vi "Photobooth.vi"() -> ()   [LabVIEW 2012]
uses:
  <vilib>/userdefined/High Color/IMAQdx.ctl
  <vilib>/LVH/i3 Twitter/Controls/Twitter Handle.ctl
  <vilib>/LVH/i3 OAuth/Controls/OAuth Handle.ctl
  <vilib>/LVH/i3 OAuth/Controls/Signature Method.ctl
  <vilib>/LVH/i3 OAuth/Controls/Credentials.ctl
  Twitter/Twitter States.ctl
  Flickr API/Flickr States.ctl
  TypeDEF/Core Data.ctl
  <vilib>/vision/Image Controls.llb/IMAQ Image.ctl
  <vilib>/LVH/i3 Twitter/SubVIs/Twitter Open - Desktop.vi
  <vilib>/LVH/i3 Twitter/Tweets with Media/Post Media Tweet - From File.vi
  C:/Users/telsey/Desktop/Personal Projects/Photobooth/Flickr API/FlickrNet-3.5.0/FlickrNet.dll
  Flickr API/FlickrNet-3.5.0/FlickrNet.dll
  <vilib>/vision/driver/NI_Vision_Acquisition_Software.lvlib
  <vilib>/vision/NI_Vision_Development_Module.lvlib
  <vilib>/LVH/i3 Twitter/i3-twitter.lvlib
  <vilib>/LVH/i3 OAuth/i3-oauth.lvlib
panel:
  out "Snapshots":T1[](array[plugin-control])
  in  "Start Button":bool
  in  "Print":bool
  out "Timer":string
  out "Dial":u16(knob) max=100 scale=0.0..100.0
  out "Image":T1(plugin-control)
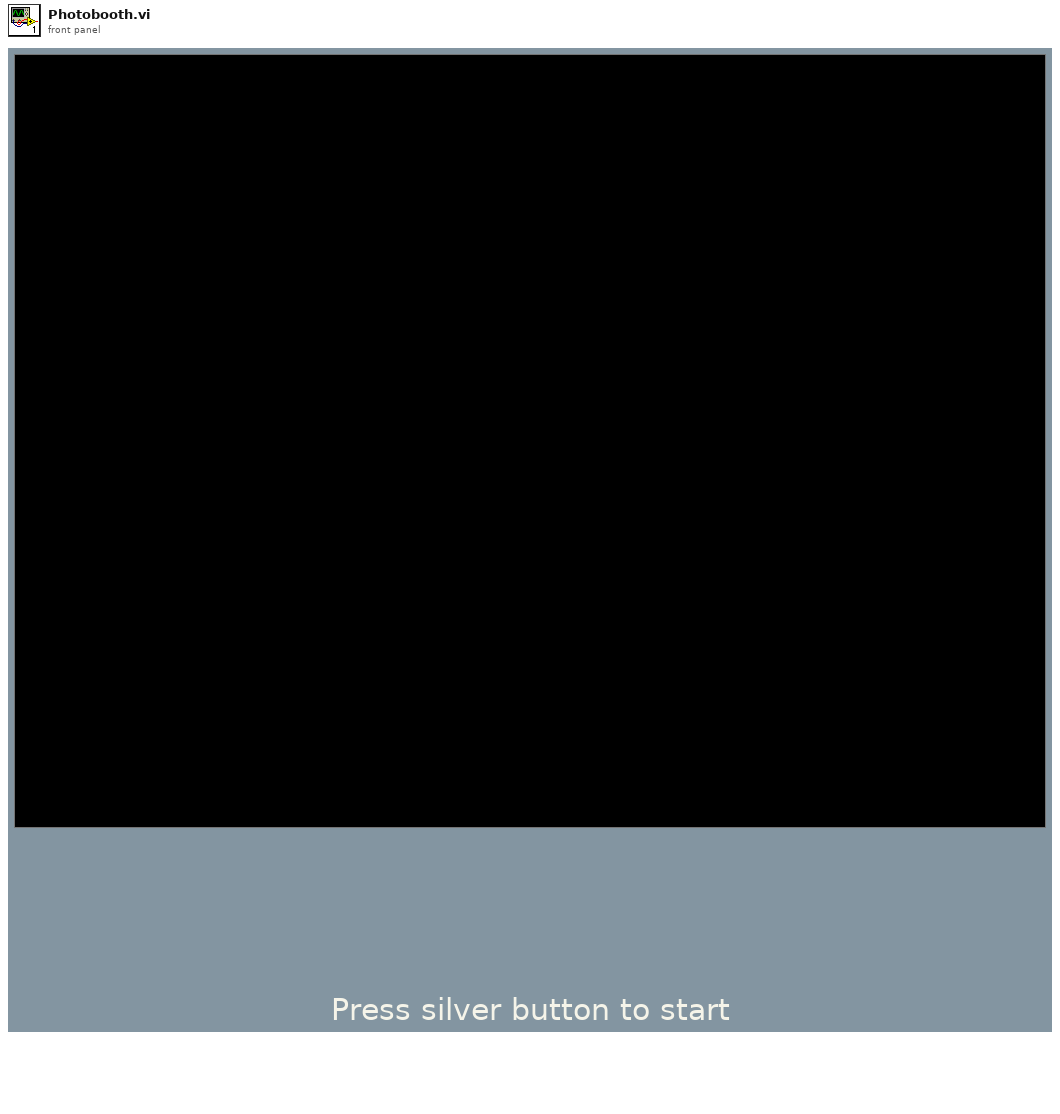
[diagram p1: front panel]
types:
  T1 = typedef "IMAQ Image.ctl" = refnum<image>
  T2 = typedef "Flickr States.ctl" = enum16{"Init", "Upload", "Close"}
  T3 = cluster{".Net Ref":refnum<k24>, "Init":cluster{"Enabled":bool, "Tag":string, "Photoset Name":string, "Photoset Description":string, "Album Cover":string}, "Path":path}
  T4 = typedef "Twitter States.ctl" = enum16{"Init", "Tweet", "Close"}
  T5 = typedef "i3-twitter.lvlib/Twitter Handle.ctl" = cluster{"OAuth Credentials":T6, "since ID":string, "max ID":string, "Screen Name":string}
  T6 = typedef "i3-oauth.lvlib/OAuth Handle.ctl" = cluster{"Signature Method":T7, "Version":string, "Client":T8, "Access":T8}
  T7 = typedef "i3-oauth.lvlib/Signature Method.ctl" = enum16{"HMAC-MD5", "HMAC-SHA1", "HMAC-SHA224", "HMAC-SHA256", "HMAC-SHA384", "HMAC-SHA512"}
  T8 = typedef "i3-oauth.lvlib/Credentials.ctl" = cluster{"Token":string, "Secret":string}
  T9 = cluster{"Handle":T5, "Access Credentials":T8, "Init":cluster{"Enabled":bool, "Tag":string}, "Image":path}
  T10 = typedef "IMAQdx.ctl" = refnum<k21>
  T11 = enum32{"invalid app kind", "Development System", "Run Time System", "Student Edition", "Embedded LabVIEW", "Evaluation", "Custom"}
  T12 = typedef "Core Data.ctl" = cluster{"Core":cluster{"Current VI Reference":refnum<vi>, "Close Panel on Exit?":bool}, "Camera":T10, "Images":T1[], "Current Image":u8, "Video Queue":refnum<queue>, "Wait":u8[], "Images Folder":path, "Photoset done":bool, "Flickr Q":refnum<queue>, "Twitter Q":refnum<queue>}
  T13 = enum32{"Invalid", "Standard", "Closed", "Hidden", "Minimized", "Maximized"}
  T14 = cluster{"Current VI Reference":refnum<vi>, "Close Panel on Exit?":bool}
  T15 = cluster{"Enabled":bool, "Tag":string, "Photoset Name":string, "Photoset Description":string, "Album Cover":string}
  T16 = cluster{"Header":path, "Image Folder":path, "Background":u32}
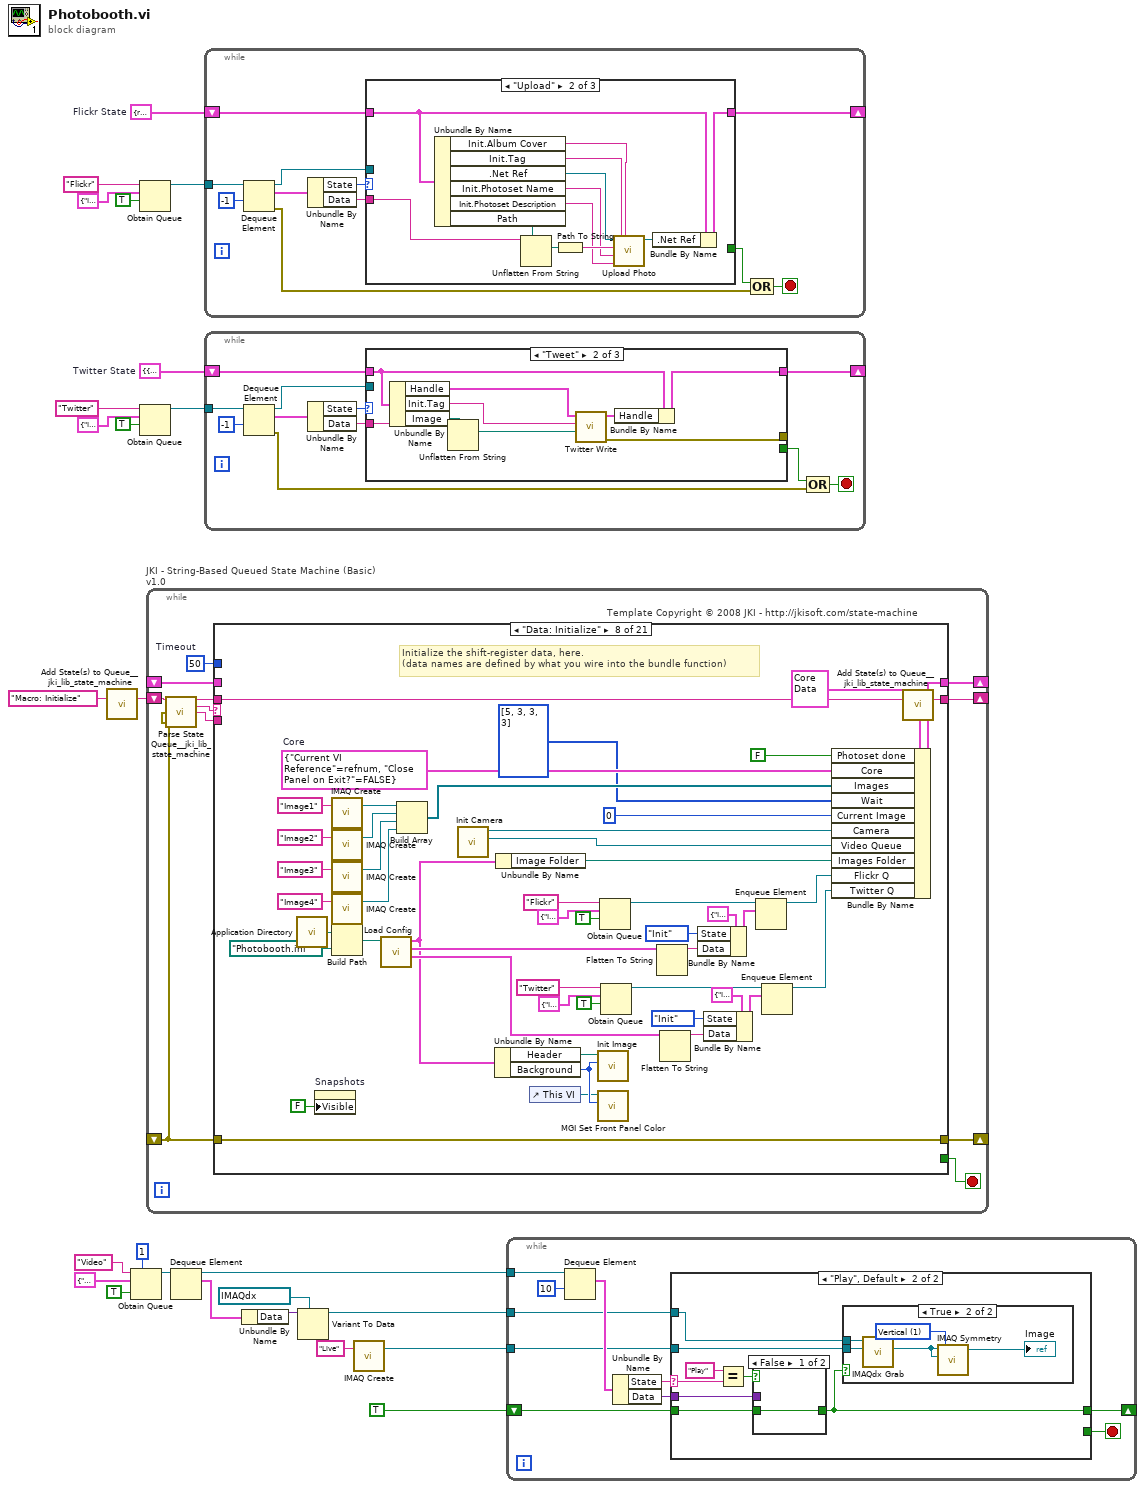
[diagram p0: block diagram]
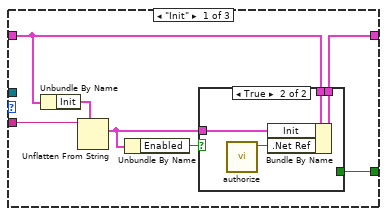
[diagram p2: hidden frame]
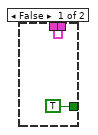
[diagram p3: hidden frame]
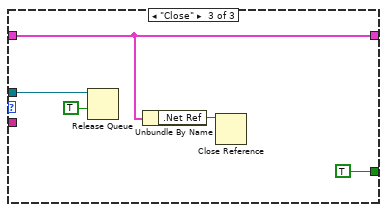
[diagram p4: hidden frame]
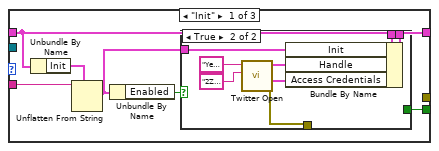
[diagram p5: hidden frame]
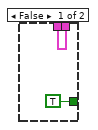
[diagram p6: hidden frame]
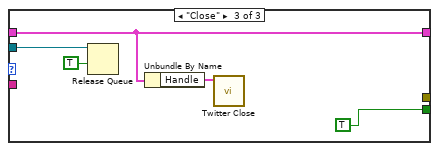
[diagram p7: hidden frame]
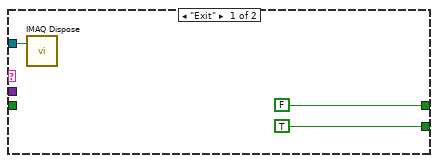
[diagram p8: hidden frame]
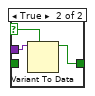
[diagram p9: hidden frame]
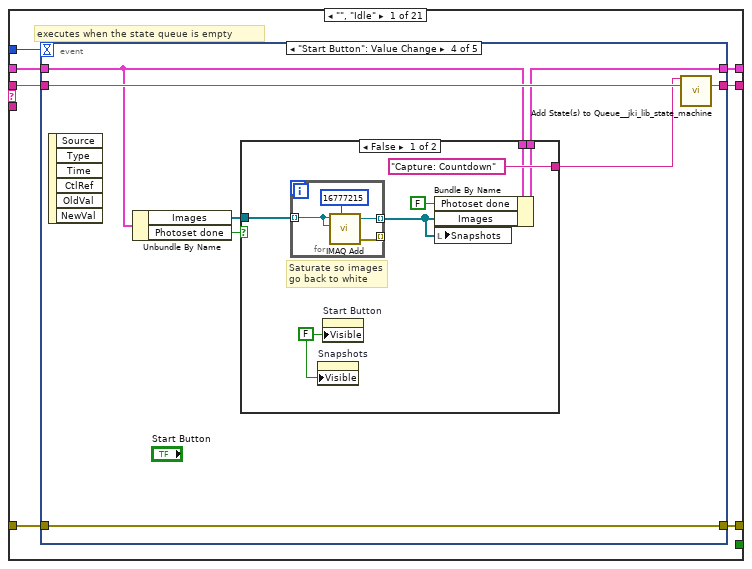
[diagram p11: hidden frame]
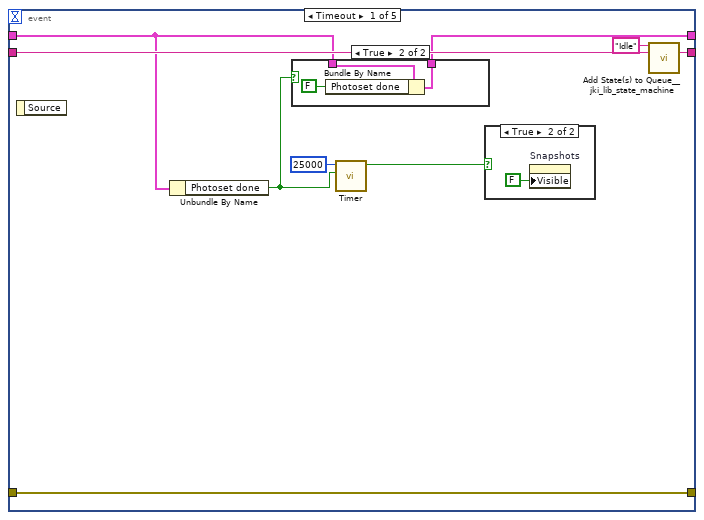
[diagram p12: hidden frame]
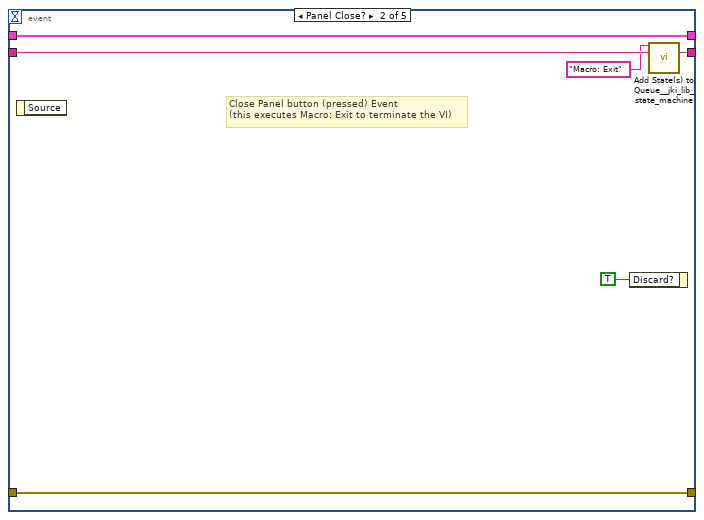
[diagram p15: hidden frame]
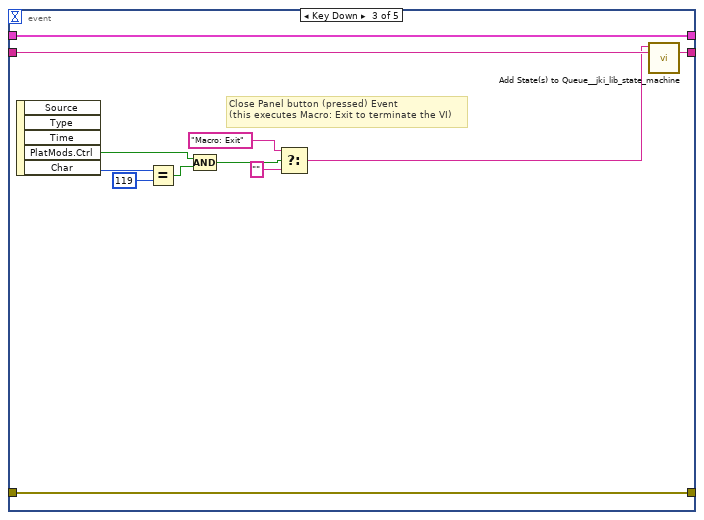
[diagram p16: hidden frame]
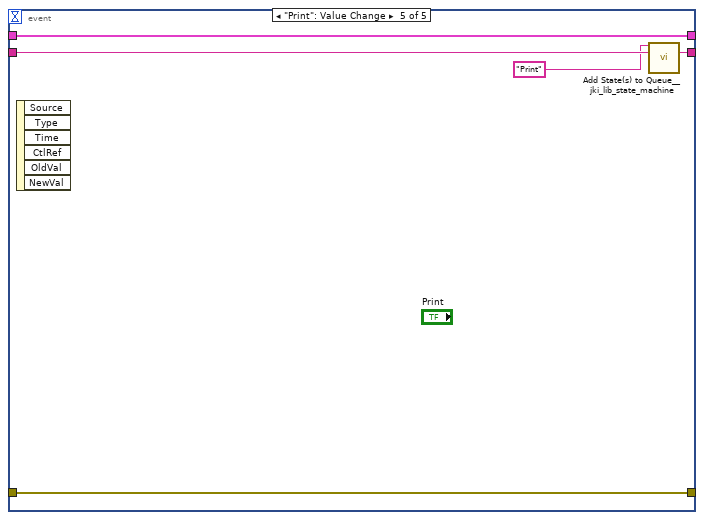
[diagram p18: hidden frame]
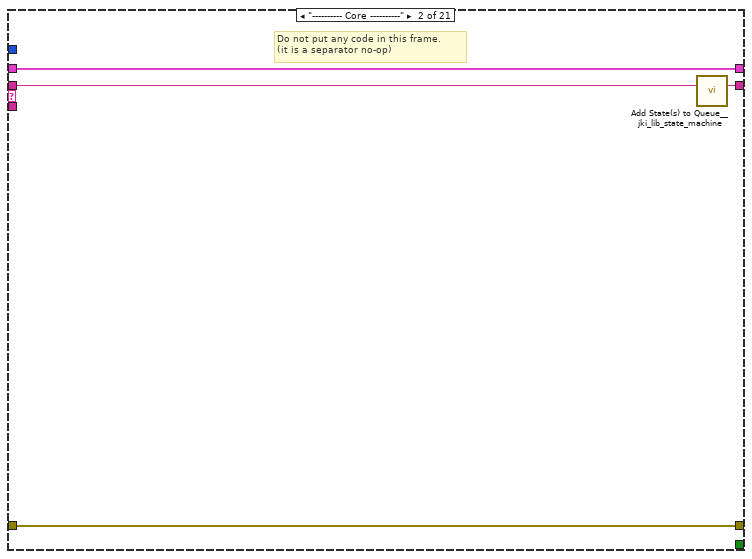
[diagram p19: hidden frame]
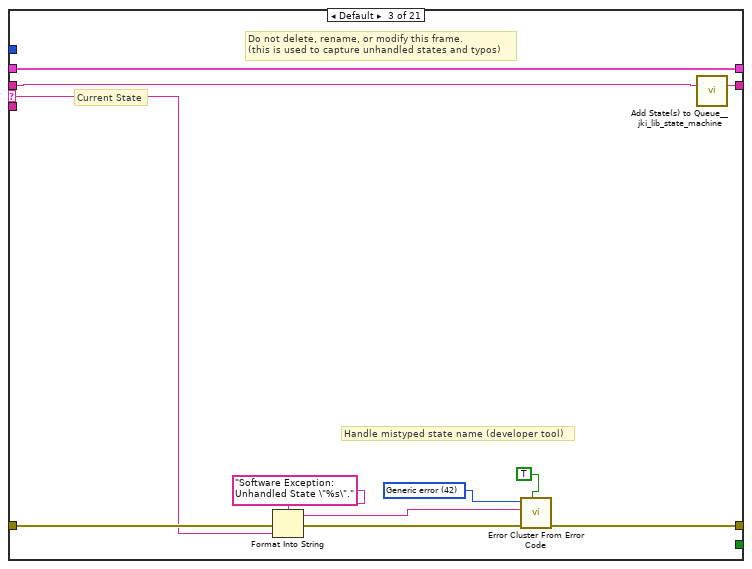
[diagram p20: hidden frame]
diagram:
  w5 = T3 {".Net Ref"=refnum, "Init"={"Enabled"=FALSE, "Tag"="", "Photoset Name"="", "Photoset Description"="", "Album Cover"=""}, "Path"=path ""}  # Flickr State
  w6 = T9 {"Handle"={"OAuth Credentials"={"Signature Method"=enum."HMAC-SHA1", "Version"="1.0", "Client"={"Token"="", "Secret"=""}, "Access"={"Token"="", "Secret"=""}}, "since ID"="", "max ID"="", "Screen Name"=""}, "Access Credentials"={"Token"="", "Secret"=""}, "Init"={"Enabled"=FALSE, "Tag"=""}, "Image"=path ""}  # Twitter State
  n1 = call <vilib>:"Add State(s) to Queue__jki_lib_state_machine.vi"("State(s) in (\"\")"="Macro: Initialize") -> ("States Out"=w25:string)  [unwired: 14 in]
  n2 = Obtain Queue(max queue size (-1, unlimited)=1, name (unnamed)="Video", element data type=cluster{"State":string, "Data":variant} {"State"="", "Data"=variant} ("State Cluster"), create if not found? (T)=TRUE) -> (queue out=w22:refnum<queue>)  [unwired: 1 in, 2 out]
  n3 = Obtain Queue(name (unnamed)="Flickr", element data type=cluster{"State":T2, "Data":string} {"State"=enum."Init", "Data"=""} ("name (unnamed)"), create if not found? (T)=TRUE) -> (queue out=w1:refnum<queue>)  [unwired: 2 in, 2 out]
  n4 = Obtain Queue(name (unnamed)="Twitter", element data type=cluster{"State":T4, "Data":string} {"State"=enum."Init", "Data"=""} ("name (unnamed)"), create if not found? (T)=TRUE) -> (queue out=w10:refnum<queue>)  [unwired: 2 in, 2 out]
  n5 = while "JKI - String-Based Queued State Machine (Basic) v1.0" {
    shift-right: [w29] -> _
    shift-left: _ -> [w28]
    shift-right: [w32] -> _
    shift-left: _ -> [w26]
    shift-right: [w31] -> _
    shift-left: w25 -> [w33]
    stop <- w30 stop-if-true
    w27 = 50  # Timeout
    # "Template Copyright © 2008 JKI - http://jkisoft.com/state-machine"
    n6 = call <vilib>:"Parse State Queue__jki_lib_state_machine.vi"("State Queue"=w33, "Error In (no error)"=w26) -> ("Remaining States"=w35:string, "Current State"=w36:string, "Arguments"=w34:string)  [unwired: 11 in]
    n7 = case shown="\"Data: Initialize\"" w36 {
      selector: w36 -> [_ _ w105 _ _ _ _ _ _ _ _ _ _ _ _ _ _ _ _ _ _]
      tunnel: w35 -> [w43 w104 w109 w127 w133 w138 w142 w191 w215 w224 w235 w241 w252 w278 w283 w293 w297 w315 w326 w350 w382]
      tunnel: w34 -> [_ _ _ _ _ _ _ _ _ _ _ w236 w246 _ _ _ _ _ _ _ _]
      tunnel: w28 -> [w41 w101 w107 w118 w130 w136 w139 _ w211 w221 w226 w239 w248 w275 w280 w290 w294 w310 w323 w343 w378]
      tunnel: [w40 w102 w111 w124 errorcluster {"status"=FALSE, "code"=0, "source"=""} ("error out") w135 w140 w188 w212 w222 w233 w237 w249 w276 w281 w291 w295 w313 w324 w348 w380] -> w32
      tunnel: w26 -> [w39 w102 w110 w124 w129 w135 w140 w188 _ w222 w233 w238 w250 w276 w281 w291 w295 w313 w324 w348 w380]
      tunnel: [w42 w103 w108 w126 w132 w137 w141 w190 w214 w223 w234 w240 w251 w277 w282 w292 w296 w314 w325 w349 w381] -> w31
      tunnel: [_ _ _ _ _ TRUE _ _ _ _ _ _ _ _ _ _ _ _ _ _ _] -> w30
      tunnel: [w38 w101 w107 w125 w130 w136 w139 w189 w211 w221 w226 w239 w248 w275 w280 w290 w294 w310 w323 w343 w377] -> w29
      tunnel: w27 -> [w37 _ _ _ _ _ _ _ _ _ _ _ _ _ _ _ _ _ _ _ _]
      frame "", "Idle" {
        # "executes when the state queue is empty"
        n8 = event shown="[3] \"Start Button\": Value Change" {
          selector: _ -> [_ _ _ _ _]
          dyn-events: _ -> [_ _ _ _ _]
          timeout: w37 -> [_ _ _ _ _]
          tunnel: w43 -> [w52 w63 w75 w83 w100]
          tunnel: [w51 w62 w74 w82 w99] -> w42
          tunnel: w41 -> [w45 w60 w72 w78 w96]
          tunnel: [w50 w61 w73 w81 w98] -> w40
          tunnel: w39 -> [w50 w61 w73 w81 w98]
          tunnel: [w44 w60 w72 w77 w96] -> w38
          event Timeout {
            n9 = event-data() -> ()  [unwired: 1 in, 1 out]
            n10 = Unbundle By Name(w45) -> ("Photoset done"=w46:bool)
            n11 = case shown="True" w46 {
              tunnel: w45 -> [w53 w56]
              tunnel: [w53 w55] -> w44
              frame False {
              }
              frame True {
                n12 = Bundle By Name(cluster=w56, "Photoset done"=FALSE) -> (w55:T12)
              }
            }
            n13 = call "Timer.vi"("Reset?"=w46, "Time Limit (ms)"=u32 25000 ("Time Limit")) -> ("Elapsed?"=w47:bool)  [unwired: 8 in, 1 out]
            n14 = case shown="True" w47 {
              frame False {
              }
              frame True {
                n15 = property on="Snapshots" class="Arr (strict)"("Visible"=FALSE) -> ()  [unwired: 2 in, 2 out]
              }
            }
            n16 = call <vilib>:"Add State(s) to Queue__jki_lib_state_machine.vi"("State(s) in Front (\"\")"="Idle" ("State(s) in Front (\"\")"), "State(s) in (\"\")"=w52) -> ("States Out"=w51:string)  [unwired: 13 in]
          }
          event Panel Close? {
            # "Close Panel button (pressed) Event\n(this executes Macro: Exit to terminate the VI)"
            n17 = event-data() -> ()  [unwired: 1 in, 1 out]
            n18 = event-data("Discard?"=TRUE) -> ()  [unwired: 1 in, 1 out]
            n19 = call <vilib>:"Add State(s) to Queue__jki_lib_state_machine.vi"("State(s) in Front (\"\")"="Macro: Exit", "State(s) in (\"\")"=w63) -> ("States Out"=w62:string)  [unwired: 13 in]
          }
          event Key Down {
            # "Close Panel button (pressed) Event\n(this executes Macro: Exit to terminate the VI)"
            n20 = event-data() -> ("PlatMods.Ctrl"=w68:bool, "Char"=w71:i16)  [unwired: 1 in, 3 out]
            n21 = Equal?(x=w71, y=i16 119) -> (x = y?=w69:bool)
            n22 = Compound Arithmetic op=AND(w68, w69) -> (w67:bool)
            n23 = Select(t="Macro: Exit", s=w67, f="") -> (s? t:f=w65:string)
            n24 = call <vilib>:"Add State(s) to Queue__jki_lib_state_machine.vi"("State(s) in Front (\"\")"=w65, "State(s) in (\"\")"=w75) -> ("States Out"=w74:string)  [unwired: 13 in]
          }
          event "Start Button": Value Change {
            n25 = event-data() -> ()  [unwired: 1 in, 6 out]
            n26 = Unbundle By Name(w78) -> ("Images"=w79:T1[], "Photoset done"=w76:bool)
            n27 = case shown="False" w76 {
              tunnel: ["Capture: Countdown" _] -> w80
              tunnel: w79 -> [w89 _]
              tunnel: w78 -> [w88 w95]
              tunnel: [w87 w95] -> w77
              frame False {
                w85 = FALSE ("Visible")
                # "Saturate so images\ngo back to white"
                n28 = for {
                  tunnel: w89 -> [w94] mode=indexing
                  tunnel: [w92] -> w86 mode=indexing
                  tunnel: [w91] -> _ mode=indexing
                  n29 = call "IMAQ Add"("Image Src A"=w94, "Constant"=16777215, "Image Dst"=w94) -> ("Image Dst Out"=w92:T1, "error out"=w91:errorcluster)  [unwired: 4 in]
                }
                n30 = property on="Snapshots" class="Arr (strict)"("Visible"=w85) -> ()  [unwired: 2 in, 2 out]
                n31 = property on="Start Button" class="Bool"("Visible"=w85) -> ()  [unwired: 2 in, 2 out]
                n32 = Bundle By Name(cluster=w88, "Photoset done"=FALSE, "Images"=w86) -> (w87:T12)
                n33 = local write "Snapshots"(w86) -> ()
              }
              frame True {
              }
            }
            n34 = call <vilib>:"Add State(s) to Queue__jki_lib_state_machine.vi"("State(s) in Front (\"\")"=w80, "State(s) in (\"\")"=w83) -> ("States Out"=w82:string)  [unwired: 13 in]
          }
          event "Print": Value Change {
            n35 = event-data() -> ()  [unwired: 1 in, 6 out]
            n36 = call <vilib>:"Add State(s) to Queue__jki_lib_state_machine.vi"("State(s) in Front (\"\")"="Print", "State(s) in (\"\")"=w100) -> ("States Out"=w99:string)  [unwired: 13 in]
          }
        }
      }
      frame "---------- Core ----------" {
        # "Do not put any code in this frame.\n(it is a separator no-op)"
        n37 = call <vilib>:"Add State(s) to Queue__jki_lib_state_machine.vi"("State(s) in (\"\")"=w104) -> ("States Out"=w103:string)  [unwired: 14 in]
      }
      frame Default {
        w114 = 42 items=["No error", "Argument error", "Memory is full", "Out of zone", "End of file", "File already open", "Generic file I/O error", "File not found", "File permission error", "Disk is full", "Duplicate path", "Too many files open", "System feature not enabled", "Resource file not found", "Cannot add resource", "Resource not found", "Image not found", "Image memory error", "Pen does not exist", "Config type invalid", "Config token not found", "Config parse error", "Config memory error", "Bad external code format", "Bad external code offset", "External code not present", "Null window", "Destroy window error", "Null menu", "Print aborted", "Bad print record", "Print driver error", "Windows error during printing", "Memory error during printing", "Print dialog error", "Generic print error", "Invalid device refnum", "Device not found", "Device parameter error", "Device unit error", "Cannot open device", "Device call aborted", "Generic error", "Cancelled by user", "Object ID too low", "Object ID too high", "Object not in heap", "Unknown heap", "Unknown object (invalid DefProc)", "Unknown object (DefProc not in table)", "Message out of range", "Invalid (null) method", "Unknown message", "Manager call not supported", "Bad address", "Network operation in progress", "Network operation timed out", "Connection is busy", "Network attribute not supported", "Network error", "Address in use", "System out of memory", "Connection aborted", "Connection refused", "Not connected", "Already connected", "Connection closed", "Initialization error (interapplication manager)", "Bad occurrence", "Wait on unbound occurrence handler", "Occurrence queue overflow", "Datalog type conflict", "Unused", "Unrecognized type (interapplication manager)", "Memory corrupt", "Failed to make temporary DLL", "Old CIN version", "Drag socket not found", "Failed to load drop-object", "Failed to register OLE object", "Failed to release OLE object", "Format specifier type mismatch", "Unknown format specifier", "Too few format specifiers", "Too many format specifiers", "Scan failed", "Newer CIN version", "Error converting to variant", "Runtime menu error", "Password tampered", "Variant attribute not found", "Incompatible variant data type", "Event data is not available", "Event Store is not present", "Occurrence is not found", "Event Queue is not created", "Event info is not available", "Refnum passed is NULL", "Error retrieving Class GUID", "Error retrieving CoClass GUID", "Error retrieving TypeLib GUID.", "Bad built application magic bytes.", "Specific driver is different from the specific driver associated with the Logical Name.", "There is no session opened to the class driver.", "Max Error", "MAX - Error with config objects", "MAX - Error loading configuration", "MAX - Group not supported"]
        # "Current State"
        # "Do not delete, rename, or modify this frame.\n(this is used to capture unhandled states and typos)"
        # "Handle mistyped state name (developer tool)"
        n38 = Format Into String(format string="Software Exception: Unhandled State \"%s\"." ("message"), error in=w110, w105) -> (resulting string=w113:string, error out=w112:errorcluster)  [unwired: 1 in]
        n39 = call <vilib>:"Error Cluster From Error Code.vi"("show call chain? (False)"=TRUE, "error in (no error)"=w112, "error message (\"\")"=w113, "error code (0)"=w114) -> ("error out"=w111:errorcluster)  [unwired: 5 in]
        n40 = call <vilib>:"Add State(s) to Queue__jki_lib_state_machine.vi"("State(s) in (\"\")"=w109) -> ("States Out"=w108:string)  [unwired: 14 in]
      }
      frame "Initialize Core Data" {
        # "Do not delete, rename, or modify this frame.\n(this is used to determine panel behavior on exit)"
        # "originally closed?"
        # "exe?"
        # "If panel starts closed or is an EXE, then close it when we exit"
        n41 = property class="App"() -> ("App.Kind"=w122:T11)  [unwired: 2 in, 2 out]
        n42 = property class="VI"() -> ("Front Panel.Open"=w123:bool)  [unwired: 2 in, 2 out]
        n43 = control-ref of="Current VI Reference"() -> (w116:refnum<vi>)
        n44 = Not(x=w123) -> (.not. x?=w120:bool)
        n45 = Equal?(x=w122, y=T11."Run Time System" ("Application:Kind")) -> (x = y?=w119:bool)
        n46 = Or(x=w120, y=w119) -> (x .or. y?=w117:bool)
        n47 = Bundle By Name(cluster=w118, "Core.Current VI Reference"=w116, "Core.Close Panel on Exit?"=w117) -> (w125:T12)
        n48 = call <vilib>:"Add State(s) to Queue__jki_lib_state_machine.vi"("State(s) in (\"\")"=w127) -> ("States Out"=w126:string)  [unwired: 14 in]
      }
      frame "Error Handler" {
        # "Unhandled Error -- Display it"
        # "Handle any errors here.\nYou can also output any states to clean-up after errors occur"
        # "Clear error"
        n49 = call <vilib>:"General Error Handler.vi"("error in (no error)"=w129) -> ()  [unwired: 10 in, 5 out]
        n50 = call <vilib>:"Add State(s) to Queue__jki_lib_state_machine.vi"("State(s) in Front (\"\")"="/* Post Error States", "State(s) in (\"\")"=w133) -> ("States Out"=w132:string)  [unwired: 13 in]
      }
      frame "Exit" {
        # "Do not put any code in this frame.\n(No errors that occur here will be handled.)"
        n51 = call <vilib>:"Add State(s) to Queue__jki_lib_state_machine.vi"("State(s) in (\"\")"=w138) -> ("States Out"=w137:string)  [unwired: 14 in]
      }
      frame "---------- Data ----------" {
        # "Do not put any code in this frame.\n(It is a separator no-op. You can make a copy of this frame to create a new Data frame)"
        n52 = call <vilib>:"Add State(s) to Queue__jki_lib_state_machine.vi"("State(s) in (\"\")"=w142) -> ("States Out"=w141:string)  [unwired: 14 in]
      }
      frame "Data: Initialize" {
        w187 = T14 {"Current VI Reference"=refnum, "Close Panel on Exit?"=FALSE}  # Core
        # "Initialize the shift-register data, here.\n(data names are defined by what you wire into the bundle function)"
        n53 = call <vilib>:"Application Directory.vi"() -> ("Application Directory"=w149:path)
        n54 = property on="Snapshots" class="Arr (strict)"("Visible"=FALSE) -> ()  [unwired: 2 in, 2 out]
        n55 = call "IMAQ Create"("Image Name"="Image1") -> ("New Image"=w186:T1)  [unwired: 4 in, 1 out]
        n56 = call "IMAQ Create"("Image Name"="Image2") -> ("New Image"=w185:T1)  [unwired: 4 in, 1 out]
        n57 = call "IMAQ Create"("Image Name"="Image3") -> ("New Image"=w184:T1)  [unwired: 4 in, 1 out]
        n58 = call "IMAQ Create"("Image Name"="Image4") -> ("New Image"=w183:T1)  [unwired: 4 in, 1 out]
        n59 = Build Path(base path=w149, name or relative path=path "Photobooth.ini" ("configuration file path")) -> (appended path=w147:path)
        n60 = call "Load Config.vi"("Config Path"=w147) -> ("Twitter"=w158:cluster{"Enabled":bool, "Tag":string}, "Flickr"=w159:T15, "Photobooth"=w146:T16)  [unwired: 8 in]
        n61 = Build Array(w186, w185, w184, w183) -> (w178:T1[])
        n62 = call "Init Camera.vi"() -> ("Video Q out"=w175:refnum<queue>, "Camera out"=w174:T10)  [unwired: 10 in]
        n63 = Unbundle By Name(w146) -> ("Header"=w145:path, "Background"=w144:u32)
        n64 = Unbundle By Name(w146) -> ("Image Folder"=w160:path)
        n65 = control-ref of="This VI"() -> (w143:refnum<vi>)
        n66 = call "Init Image.vi"("Pane Color"=w144, "Header Path"=w145) -> ()  [unwired: 10 in]
        n67 = call <userlib>:"MGI Set Front Panel Color.vi"("Color (System Panel)"=w144, "VI Reference In (Caller)"=w143) -> ()  [unwired: 7 in, 2 out]
        n68 = Obtain Queue(name (unnamed)="Flickr", element data type=cluster{"State":T2, "Data":string} {"State"=enum."Init", "Data"=""} ("name (unnamed)"), create if not found? (T)=TRUE) -> (queue out=w163:refnum<queue>)  [unwired: 2 in, 2 out]
        n69 = Obtain Queue(name (unnamed)="Twitter", element data type=cluster{"State":T4, "Data":string} {"State"=enum."Init", "Data"=""} ("name (unnamed)"), create if not found? (T)=TRUE) -> (queue out=w167:refnum<queue>)  [unwired: 2 in, 2 out]
        n70 = Flatten To String(anything=w159) -> (data string=w154:string)  [unwired: 3 in, 2 out]
        n71 = Flatten To String(anything=w158) -> (data string=w150:string)  [unwired: 3 in, 2 out]
        n72 = Bundle By Name(cluster=cluster{"State":T2, "Data":string} {"State"=enum."Init", "Data"=""} ("name (unnamed)"), "State"=Flickr_States."Init", "Data"=w154) -> (w156:cluster{"State":T2, "Data":string})
        n73 = Bundle By Name(cluster=cluster{"State":T4, "Data":string} {"State"=enum."Init", "Data"=""} ("element"), "State"=Twitter_States."Init", "Data"=w150) -> (w152:cluster{"State":T4, "Data":string})
        n74 = Enqueue Element(queue=w163, element=w156) -> (queue out=w161:refnum<queue>)  [unwired: 2 in, 2 out]
        n75 = Enqueue Element(queue=w167, element=w152) -> (queue out=w166:refnum<queue>)  [unwired: 2 in, 2 out]
        n76 = Bundle By Name(cluster=T12 {"Core"={"Current VI Reference"=refnum, "Close Panel on Exit?"=FALSE}, "Camera"="", "Images"=[], "Current Image"=0, "Video Queue"=refnum, "Wait"=[], "Images Folder"=path "", "Photoset done"=FALSE, "Flickr Q"=refnum, "Twitter Q"=refnum}, "Photoset done"=FALSE, "Core"=w187, "Images"=w178, "Wait"=u8[] [5, 3, 3, 3], "Current Image"=u8 0, "Camera"=w174, "Video Queue"=w175, "Images Folder"=w160, "Flickr Q"=w161, "Twitter Q"=w166) -> (w189:T12)
        n77 = call <vilib>:"Add State(s) to Queue__jki_lib_state_machine.vi"("State(s) in (\"\")"=w191) -> ("States Out"=w190:string)  [unwired: 14 in]
      }
      frame "Data: Cleanup" {
        # "This loop runs to make sure the bottom loop processes\nthe Exit command before the camera is closed so the \nvideo acquisition does not error"
        # "Cleanup any data and references, here.\n(this is called automatically, by the Macro: Exit)"
        n78 = Unbundle By Name(w211) -> ("Twitter Q"=w195:refnum<queue>, "Flickr Q"=w199:refnum<queue>, "Core.Current VI Reference"=w213:refnum<vi>, "Images"=w210:T1[], "Camera"=w201:T10, "Video Queue"=w205:refnum<queue>)
        n79 = Bundle By Name(cluster=cluster{"State":string, "Data":variant} {"State"="", "Data"=variant} ("element"), "State"="Exit") -> (w207:cluster{"State":string, "Data":variant})
        n80 = Enqueue Element(queue=w205, element=w207) -> (queue out=w204:refnum<queue>)  [unwired: 2 in, 2 out]
        n81 = while {
          shift-right: [w216] -> w203
          shift-left: w204 -> [w217]
          stop <- w218 stop-if-true
          n82 = Get Queue Status(queue=w217) -> (queue out=w216:refnum<queue>, # elements in queue=w219:i32)  [unwired: 2 in, 6 out]
          n83 = Equal To 0?(x=w219) -> (x = 0?=w218:bool)
        }
        n84 = Bundle By Name(cluster=cluster{"State":T4, "Data":string} {"State"=enum."Init", "Data"=""} ("element"), "State"=Twitter_States."Close") -> (w197:cluster{"State":T4, "Data":string})
        n85 = Bundle By Name(cluster=cluster{"State":T2, "Data":string} {"State"=enum."Init", "Data"=""} ("element"), "State"=Flickr_States."Close") -> (w193:cluster{"State":T2, "Data":string})
        n86 = Enqueue Element(queue=w195, element=w197) -> ()  [unwired: 2 in, 3 out]
        n87 = Enqueue Element(queue=w199, element=w193) -> ()  [unwired: 2 in, 3 out]
        n88 = for {
          tunnel: w210 -> [w220] mode=indexing
          n89 = call "IMAQ Dispose"("Image"=w220) -> ()  [unwired: 5 in, 1 out]
        }
        n90 = Release Queue(queue=w203, force destroy? (F)=TRUE) -> (error out=w202:errorcluster)  [unwired: 1 in, 2 out]
        n91 = call <vilib>:"IMAQdx Close Camera.vi"("error in"=w202, "Session In"=w201) -> ("error out"=w200:errorcluster)  [unwired: 9 in]
        n92 = Close Reference(reference=w213, error in (no error)=w200) -> (error out=w212:errorcluster)
        n93 = call <vilib>:"Add State(s) to Queue__jki_lib_state_machine.vi"("State(s) in (\"\")"=w215) -> ("States Out"=w214:string)  [unwired: 14 in]
      }
      frame "---------- UI ----------" {
        # "Do not put any code in this frame.\n(It is a separator no-op. You can make a copy of this frame to create a new UI frame)"
        n94 = call <vilib>:"Add State(s) to Queue__jki_lib_state_machine.vi"("State(s) in (\"\")"=w224) -> ("States Out"=w223:string)  [unwired: 14 in]
      }
      frame "UI: Initialize" {
        w231 = FALSE ("Visible")
        # "Initialize the User Interface, here.\n(this is called automatically, by the Macro: Init)"
        n95 = Unbundle By Name(w226) -> ("Wait"=w230:u8[])
        n96 = Index Array(array=w230) -> (element=w227:u8)  [unwired: 1 in]
        n97 = Number To Decimal String(number=w227) -> (decimal integer string=w229:string)  [unwired: 1 in]
        n98 = property on="Dial" class="Knob (strict)"("Value"=u16 0 ("Dial"), "Visible"=w231) -> ()  [unwired: 2 in, 2 out]
        n99 = property on="Timer" class="Str"("Visible"=w231, "Value"=w229) -> ()  [unwired: 2 in, 2 out]
        n100 = property on="Start Button" class="Bool"("Visible"=TRUE) -> ()  [unwired: 2 in, 2 out]
        n101 = property on="Snapshots" class="Arr (strict)"("Visible"=FALSE) -> ()  [unwired: 2 in, 2 out]
        n102 = call <vilib>:"Add State(s) to Queue__jki_lib_state_machine.vi"("State(s) in (\"\")"=w235) -> ("States Out"=w234:string)  [unwired: 14 in]
      }
      frame "UI: Cursor Set" {
        # "Argument"
        # "Set and Unset Cursor Busy.\n(Usage: \"UI: Cursor Set >> Busy|Idle\")"
        n103 = case shown="\"Idle\", Default" w236 {
          tunnel: w238 -> [w243 w245]
          tunnel: [w242 w244] -> w237
          frame "Idle", Default {
            n104 = call <vilib>:"Unset Busy.vi"("error in (no error)"=w243) -> ("error out"=w242:errorcluster)  [unwired: 10 in]
          }
          frame "Busy" {
            n105 = call <vilib>:"Set Busy.vi"("error in (no error)"=w245) -> ("error out"=w244:errorcluster)  [unwired: 9 in, 1 out]
          }
        }
        n106 = call <vilib>:"Add State(s) to Queue__jki_lib_state_machine.vi"("State(s) in (\"\")"=w241) -> ("States Out"=w240:string)  [unwired: 14 in]
      }
      frame "UI: Front Panel State" {
        # "Argument"
        # "Set Front Panel Open or Closed\n(Usage: \"UI: Front Panel State >> Open|Close\")"
        n107 = Unbundle By Name(w248) -> ("Core.Current VI Reference"=w247:refnum<vi>)
        n108 = case shown="\"Close\"" w246 {
          tunnel: w250 -> [w256 w269]
          tunnel: [w258 w270] -> w249
          tunnel: w247 -> [w257 w267]
          frame "Open", Default {
            n109 = property class="VI"(reference=w257, error in=w256) -> (reference out=w254:refnum<vi>, error out=w255:errorcluster, "Front Panel.Open"=w253:bool)
            n110 = case shown="False" w253 {
              tunnel: [w261 w264] -> w258
              tunnel: w255 -> [w260 w264]
              tunnel: w254 -> [w259 _]
              frame False {
                n111 = invoke class="VI" method="FP.Open"(reference=w259, error in=w260, "Activate"=TRUE, "State"=T13."Standard") -> (error out=w261:errorcluster)  [unwired: 1 in, 4 out]
              }
              frame True {
              }
            }
          }
          frame "Close" {
            n112 = property class="VI"(reference=w267, error in=w269) -> (reference out=w266:refnum<vi>, error out=w268:errorcluster, "Front Panel.Open"=w265:bool)
            n113 = case shown="False" w265 {
              tunnel: [w271 w274] -> w270
              tunnel: w268 -> [w271 w273]
              tunnel: w266 -> [_ w272]
              frame False {
              }
              frame True {
                n114 = invoke class="VI" method="FP.Close"(reference=w272, error in=w273) -> (error out=w274:errorcluster)  [unwired: 1 in, 2 out]
              }
            }
          }
        }
        n115 = call <vilib>:"Add State(s) to Queue__jki_lib_state_machine.vi"("State(s) in (\"\")"=w252) -> ("States Out"=w251:string)  [unwired: 14 in]
      }
      frame "---------- Macro ----------" {
        # "Do not put any code in this frame.\n(It is a separator no-op. You can make a copy of this frame to create a new Macro frame)"
        n116 = call <vilib>:"Add State(s) to Queue__jki_lib_state_machine.vi"("State(s) in (\"\")"=w278) -> ("States Out"=w277:string)  [unwired: 14 in]
      }
      frame "Macro: Initialize" {
        w279 = "Data: Initialize\nInitialize Core Data\nUI: Initialize\nUI: Front Panel State >> Open\nIdle"  # Data: Initialize Initialize Core Data UI: Initialize UI: Front Panel State >> Open Idle
        # "Initialization Macro\n(This is called once, when the VI starts)"
        n117 = call <vilib>:"Add State(s) to Queue__jki_lib_state_machine.vi"("State(s) in Front (\"\")"=w279, "State(s) in (\"\")"=w283) -> ("States Out"=w282:string)  [unwired: 13 in]
      }
      frame "Macro: Exit" {
        # "Exit Macro\n(This is called once, when the VI exits)"
        n118 = Unbundle By Name(w290) -> ("Core.Close Panel on Exit?"=w289:bool)
        n119 = Select(t="UI: Front Panel State >> Close", s=w289, f="") -> (s? t:f=w286:string)
        n120 = call <vilib>:"Add State(s) to Queue__jki_lib_state_machine.vi"("State(s) in (\"\")"=w286, "State(s) at Back (\"\")"="Data: Cleanup\nExit") -> ("States Out"=w284:string)  [unwired: 13 in]
        n121 = call <vilib>:"Add State(s) to Queue__jki_lib_state_machine.vi"("State(s) in Front (\"\")"=w284, "State(s) in (\"\")"=w293) -> ("States Out"=w292:string)  [unwired: 13 in]
      }
      frame "---------- Capture ----------" {
        # "Template Separator\n(You can make a copy of, or modify, this frame)"
        n122 = call <vilib>:"Add State(s) to Queue__jki_lib_state_machine.vi"("State(s) in (\"\")"=w297) -> ("States Out"=w296:string)  [unwired: 14 in]
      }
      frame "Print" {
        # "Print\nSend Images to Print Sheet"
        n123 = Unbundle By Name(w310) -> ("Flickr Q"=w299:refnum<queue>, "Images Folder"=w300:path, "Images"=w312:T1[], "Twitter Q"=w298:refnum<queue>)
        n124 = call "Print Image.vi"("Images"=w312, "Path"=w300) -> ("New Image Path"=w305:path)  [unwired: 9 in]
        n125 = Flatten To String(anything=w305) -> (data string=w306:string)  [unwired: 3 in, 2 out]
        n126 = Flatten To String(anything=w305) -> (data string=w302:string)  [unwired: 3 in, 2 out]
        n127 = Bundle By Name(cluster=cluster{"State":T2, "Data":string} {"State"=enum."Init", "Data"=""} ("element"), "State"=Flickr_States."Upload", "Data"=w306) -> (w308:cluster{"State":T2, "Data":string})
        n128 = Bundle By Name(cluster=cluster{"State":T4, "Data":string} {"State"=enum."Init", "Data"=""} ("element"), "State"=Twitter_States."Tweet", "Data"=w302) -> (w301:cluster{"State":T4, "Data":string})
        n129 = Enqueue Element(queue=w299, element=w308) -> ()  [unwired: 2 in, 3 out]
        n130 = Enqueue Element(queue=w298, element=w301) -> ()  [unwired: 2 in, 3 out]
        n131 = call <vilib>:"Add State(s) to Queue__jki_lib_state_machine.vi"("State(s) in Front (\"\")"="Idle" ("State(s) in Front (\"\")"), "State(s) in (\"\")"=w315) -> ("States Out"=w314:string)  [unwired: 13 in]
      }
      frame "Capture: Countdown" {
        # "Your code here.\n(You can make a copy of, or modify, this frame)"
        n132 = Unbundle By Name(w323) -> ("Wait"=w318:u8[], "Current Image"=w317:u8, "Images"=w322:T1[])
        n133 = Array Size(array=w322) -> (size(s)=w321:i32)
        n134 = Index Array(array=w318, index=w317) -> (element=w316:u8)
        n135 = Less?(x=w317, y=w321) -> (x < y?=w320:bool)
        n136 = case shown="True" w320 {
          tunnel: w316 -> [_ w329]
          tunnel: ["Update Images" "Capture: Image"] -> w319
          frame False {
          }
          frame True {
            w331 = TRUE ("Visible")
            w328 = 100 ("y")
            n137 = property on="Dial" class="Knob (strict)"("Value"=u16 0 ("Dial"), "Visible"=w331) -> (error out=w330:errorcluster)  [unwired: 2 in, 1 out]
            n138 = property on="Timer" class="Str"("Visible"=w331) -> ()  [unwired: 2 in, 2 out]
            n139 = Multiply(x=w328, y=w329) -> (x*y=w333:i32)
            n140 = for {
              N: w333 -> [_]
              tunnel: w330 -> [_]
              tunnel: w329 -> [w337]
              tunnel: w328 -> [w335]
              i -> [w340]
              n141 = Quotient & Remainder(x=w340, y=w335) -> (x-y*floor(x/y)=→"Dial":i32, floor(x/y)=w336:i32)
              n142 = Wait (ms)(milliseconds to wait=u32 10) -> ()  [unwired: 1 out]
              n143 = Compound Arithmetic op=ADD(invert w336, w337) -> (w338:i32)
              n144 = Number To Decimal String(number=w338) -> (decimal integer string=→"Timer":string)  [unwired: 1 in]
            }
          }
        }
        n145 = call <vilib>:"Add State(s) to Queue__jki_lib_state_machine.vi"("State(s) in Front (\"\")"=w319, "State(s) in (\"\")"=w326) -> ("States Out"=w325:string)  [unwired: 13 in]
      }
      frame "Capture: Image" {
        w344 = FALSE ("Visible")
        # "Your code here.\n(You can make a copy of, or modify, this frame)"
        n146 = Wait (ms)(milliseconds to wait=u32 150) -> (millisecond timer value=w345:u32)
        n147 = property on="Dial" class="Knob (strict)"("Visible"=w344) -> ()  [unwired: 2 in, 2 out]
        n148 = property on="Timer" class="Str"("Visible"=w344) -> ()  [unwired: 2 in, 2 out]
        n149 = flat-sequence {
          tunnel: w343 -> [w351]
          tunnel: w345 -> [_]
          frame #0 {
            n150 = Unbundle By Name(w351) -> ("Camera"=w361:T10, "Images"=w353:T1[], "Current Image"=w352:u8, "Video Queue"=w359:refnum<queue>)
            n151 = Bundle By Name(cluster=cluster{"State":string, "Data":variant} {"State"="", "Data"=variant} ("element"), "State"="Play", "Data"=FALSE) -> (w357:cluster{"State":string, "Data":variant})
            n152 = Index Array(array=w353, index=w352) -> (element=w360:T1)
            n153 = Enqueue Element(queue=w359, element=w357) -> (error out=w354:errorcluster)  [unwired: 2 in, 2 out]
            n154 = call <vilib>:"IMAQdx Grab.vi"("error in"=w354, "Image In"=w360, "Session In"=w361) -> ()  [unwired: 5 in, 4 out]
          }
        }
        n155 = call <vilib>:"Add State(s) to Queue__jki_lib_state_machine.vi"("State(s) in Front (\"\")"="Update Images" ("State(s) in Front (\"\")"), "State(s) in (\"\")"=w350) -> ("States Out"=w349:string)  [unwired: 13 in]
      }
      frame "Update Images" {
        # "Update Timer so user doesn't\nsee 1 before timer starts"
        # "Your code here.\n(You can make a copy of, or modify, this frame)"
        n156 = flat-sequence {
          tunnel: w372 -> [w384]
          frame #0 {
            n157 = Wait (ms)(milliseconds to wait=u32 1500) -> ()  [unwired: 1 out]
          }
          frame #1 {
            n158 = Bundle By Name(cluster=cluster{"State":string, "Data":variant} {"State"="", "Data"=variant} ("element"), "State"="Play", "Data"=TRUE) -> (w387:cluster{"State":string, "Data":variant})
            n159 = Enqueue Element(queue=w384, element=w387) -> ()  [unwired: 2 in, 3 out]
          }
        }
        n160 = Unbundle By Name(w378) -> ("Wait"=w366:u8[], "Current Image"=w379:u8, "Images"=w376:T1[], "Video Queue"=w372:refnum<queue>)
        "Snapshots" <- w376
        n161 = Array Size(array=w376) -> (size(s)=w371:i32)
        n162 = Increment(x=w379) -> (x+1=w364:u8)
        n163 = Quotient & Remainder(x=w364, y=w371) -> (x-y*floor(x/y)=w368:i32)  [unwired: 1 out]
        n164 = Less?(x=w364, y=w371) -> (x < y?=w370:bool)
        n165 = Index Array(array=w366, index=w368) -> (element=w367:u8)
        n166 = Bundle By Name(cluster=w378, "Photoset done"=TRUE, "Current Image"=w368) -> (w377:T12)
        n167 = property on="Snapshots" class="Arr (strict)"("Number of Columns"=w364, "Visible"=TRUE) -> ()  [unwired: 2 in, 2 out]
        n168 = Number To Decimal String(number=w367) -> (decimal integer string=w369:string)  [unwired: 1 in]
        n169 = Not(x=w370) -> (.not. x?=w365:bool)
        n170 = local write "Timer"(w369) -> ()
        n171 = Select(t="Capture: Countdown", s=w370, f="Print" ("State(s) in Front (\"\")")) -> (s? t:f=w373:string)
        n172 = property on="Start Button" class="Bool"("Visible"=w365) -> ()  [unwired: 2 in, 2 out]
        n173 = call <vilib>:"Add State(s) to Queue__jki_lib_state_machine.vi"("State(s) in Front (\"\")"=w373, "State(s) in (\"\")"=w382) -> ("States Out"=w381:string)  [unwired: 13 in]
      }
    }
  }
  n174 = Dequeue Element(queue=w22) -> (queue out=w17:refnum<queue>, element=w16:cluster{"State":string, "Data":variant})  [unwired: 2 in, 2 out]
  n175 = while {
    tunnel: w1 -> [w399]
    shift-right: [w394] -> _
    shift-left: w5 -> [w396]
    stop <- w389 stop-if-true
    n176 = Dequeue Element(queue=w399, timeout in ms (-1)=-1) -> (queue out=w392:refnum<queue>, element=w397:cluster{"State":T2, "Data":string}, error out=w390:errorcluster)  [unwired: 1 in, 1 out]
    n177 = Unbundle By Name(w397) -> ("State"=w395:T2, "Data"=w393:string)
    n178 = case shown="\"Upload\"" w395 {
      tunnel: w396 -> [w404 w422 w429]
      tunnel: [w406 w421 w429] -> w394
      tunnel: w393 -> [w405 w424 _]
      tunnel: w392 -> [_ _ w427]
      tunnel: [w400 _ TRUE] -> w391
      frame "Init" {
        n179 = Unbundle By Name(w404) -> ("Init"=w403:T15)
        n180 = Unflatten From String(type=w403, binary string=w405) -> (value=w401:T15)  [unwired: 3 in, 2 out]
        n181 = Unbundle By Name(w401) -> ("Enabled"=w402:bool)
        n182 = case shown="True" w402 {
          tunnel: [w408 w412] -> w406
          tunnel: w404 -> [w408 w410]
          tunnel: w401 -> [_ w409]
          tunnel: [TRUE _] -> w400
          frame False {
          }
          frame True {
            n183 = call "authorize.vi"() -> ("Flickr Ref out"=w411:refnum<k24>)  [unwired: 11 in]
            n184 = Bundle By Name(cluster=w410, "Init"=w409, ".Net Ref"=w411) -> (w412:T3)
          }
        }
      }
      frame "Upload" {
        n185 = Unbundle By Name(w422) -> ("Init.Album Cover"=w413:string, "Init.Tag"=w418:string, ".Net Ref"=w414:refnum<k24>, "Init.Photoset Name"=w416:string, "Init.Photoset Description"=w417:string, "Path"=w423:path)
        n186 = Unflatten From String(type=w423, binary string=w424) -> (value=w415:path)  [unwired: 3 in, 2 out]
        n187 = Path To String(path=w415) -> (string=w419:string)
        n188 = call "Upload Photo.vi"("Photo tags"=w418, "Album Cover"=w413, "Description"=w417, "Photoset Name"=w416, "Image Path"=w419, "Flickr Ref"=w414) -> ("Flickr Ref out"=w420:refnum<k24>)  [unwired: 5 in]
        n189 = Bundle By Name(cluster=w422, ".Net Ref"=w420) -> (w421:T3)
      }
      frame "Close" {
        n190 = Release Queue(queue=w427, force destroy? (F)=TRUE) -> ()  [unwired: 1 in, 3 out]
        n191 = Unbundle By Name(w429) -> (".Net Ref"=w428:refnum<k24>)
        n192 = Close Reference(reference=w428) -> ()  [unwired: 1 in, 1 out]
      }
    }
    n193 = Compound Arithmetic op=OR(w391, w390) -> (w389:bool)
  }
  n194 = while {
    tunnel: w10 -> [w440]
    shift-right: [w435] -> _
    shift-left: w6 -> [w437]
    stop <- w430 stop-if-true
    n195 = Dequeue Element(queue=w440, timeout in ms (-1)=-1) -> (queue out=w433:refnum<queue>, element=w438:cluster{"State":T4, "Data":string}, error out=w431:errorcluster)  [unwired: 1 in, 1 out]
    n196 = Unbundle By Name(w438) -> ("State"=w436:T4, "Data"=w434:string)
    n197 = case shown="\"Tweet\"" w436 {
      tunnel: w437 -> [w445 w463 w471]
      tunnel: [w447 w462 w471] -> w435
      tunnel: w434 -> [w443 w466 _]
      tunnel: w433 -> [_ _ w468]
      tunnel: [w446 _ TRUE] -> w432
      tunnel: [_ w458 _] -> _
      frame "Init" {
        n198 = Unbundle By Name(w445) -> ("Init"=w444:cluster{"Enabled":bool, "Tag":string})
        n199 = Unflatten From String(type=w444, binary string=w443) -> (value=w441:cluster{"Enabled":bool, "Tag":string})  [unwired: 3 in, 2 out]
        n200 = Unbundle By Name(w441) -> ("Enabled"=w442:bool)
        n201 = case shown="True" w442 {
          tunnel: w445 -> [w449 w455]
          tunnel: [w449 w454] -> w447
          tunnel: [TRUE _] -> w446
          tunnel: [_ w451] -> _
          tunnel: w441 -> [_ w450]
          frame False {
          }
          frame True {
            n202 = call-poly <vilib>:"Twitter Open.vi"("Consumer Secret"="2ZDmzpqyNpiByDQQhohs8dSN9LtSH3nAod3QldeU", "Consumer Key"="Ye1QTjAaMzT6uHrDUqJR2w") -> ("error out"=w451:errorcluster, "Access Credentials (out)"=w452:T8, "Twitter Handle Out"=w453:T5)  [unwired: 7 in]
            n203 = Bundle By Name(cluster=w455, "Init"=w450, "Handle"=w453, "Access Credentials"=w452) -> (w454:T9)
          }
        }
      }
      frame "Tweet" {
        n204 = Unbundle By Name(w463) -> ("Handle"=w461:T5, "Init.Tag"=w459:string, "Image"=w465:path)
        n205 = Unflatten From String(type=w465, binary string=w466) -> (value=w460:path)  [unwired: 3 in, 2 out]
        n206 = call-poly <vilib>:"Twitter Write.vi"("Picture File (PNG, JPG, GIF)"=w460, "Tweet"=w459, "Twitter Handle In"=w461) -> ("error out"=w458:errorcluster, "Twitter Handle Out"=w464:T5)  [unwired: 7 in]
        n207 = Bundle By Name(cluster=w463, "Handle"=w464) -> (w462:T9)
      }
      frame "Close" {
        n208 = Release Queue(queue=w468, force destroy? (F)=TRUE) -> ()  [unwired: 1 in, 3 out]
        n209 = Unbundle By Name(w471) -> ("Handle"=w470:T5)
        n210 = call <vilib>:"Twitter Close.vi"("Twitter Handle In"=w470) -> ()  [unwired: 10 in, 1 out]
      }
    }
    n211 = Compound Arithmetic op=OR(w432, w431) -> (w430:bool)
  }
  n212 = Unbundle By Name(w16) -> ("Data"=w15:variant)
  n213 = Variant To Data(type=T10 "Logitech" ("Session In"), Variant=w15) -> (data=w11:T10)  [unwired: 1 in, 1 out]
  n214 = call "IMAQ Create"("Image Name"="Live") -> ("New Image"=w18:T1)  [unwired: 4 in, 1 out]
  n215 = while {
    tunnel: w18 -> [w475]
    tunnel: w17 -> [w481]
    tunnel: w11 -> [w476]
    shift-right: [w473] -> _
    shift-left: TRUE -> [w472]
    stop <- w477 stop-if-true
    n216 = Dequeue Element(queue=w481, timeout in ms (-1)=10) -> (element=w479:cluster{"State":string, "Data":variant})  [unwired: 1 in, 3 out]
    n217 = Unbundle By Name(w479) -> ("State"=w478:string, "Data"=w474:variant)
    n218 = case shown="\"Play\", Default" w478 {
      selector: w478 -> [_ w490]
      tunnel: [TRUE _] -> w477
      tunnel: w476 -> [_ w492]
      tunnel: w475 -> [w482 w491]
      tunnel: w474 -> [_ w487]
      tunnel: [FALSE w486] -> w473
      tunnel: w472 -> [_ w485]
      frame "Exit" {
        n219 = call "IMAQ Dispose"("Image"=w482) -> ()  [unwired: 5 in, 1 out]
      }
      frame "Play", Default {
        n220 = Equal?(x="Play" ("y"), y=w490) -> (x = y?=w488:bool)
        n221 = case shown="False" w488 {
          selector: w488 -> [_ w496]
          tunnel: w487 -> [_ w495]
          tunnel: [w493 w494] -> w486
          tunnel: w485 -> [w493 _]
          frame False {
          }
          frame True {
            n222 = Variant To Data(type=w496, Variant=w495) -> (data=w494:bool)  [unwired: 1 in, 1 out]
          }
        }
        n223 = case shown="True" w486 {
          tunnel: w491 -> [_ w501]
          tunnel: w492 -> [_ w500]
          frame False {
          }
          frame True {
            w497 = u32 1 items=["Horizontal", "Vertical", "Central", "1st Diagonal", "2nd Diagonal"] ("Type of Symmetry")
            n224 = call <vilib>:"IMAQdx Grab.vi"("Image In"=w501, "Session In"=w500) -> ("Image Out"=w498:T1)  [unwired: 6 in, 3 out]
            n225 = call "IMAQ Symmetry"("Type of Symmetry"=w497, "Image Dst"=w498, "Image Src"=w498) -> ("Image Dst Out"=→"Image":T1)  [unwired: 2 in, 1 out]
          }
        }
      }
    }
  }
